vi "Save or Load Config.vi"(2 "GUI Helper Q":refnum<queue>, 4 "Config Select Ref":refnum<vi>, 5 "Auto Clust":refnum<vi>, 6 "Task Info in":refnum<vi>, 7 "Save?":bool, 8 "error in (no error)":errorcluster, 9 "Task Configuration Name":string, 10 "Task Selection in":refnum<vi>, 11 "GUI in":refnum<class "GUI.lvclass">) -> (0 "error out":errorcluster, 3 "GUI out":refnum<class "GUI.lvclass">)   [LabVIEW 2020, in "GUI.lvlib" / "GUI.lvclass"]
uses:
  GUI.lvclass
  Task selection df.ctl
  Task info df.ctl
  Automate df.ctl
  Task Active Enum df.ctl
  GUI.lvclass/GUI.ctl
  <vilib>/Utility/config.llb/NI_LVConfig.lvlib
panel:
  # "Patterns"
  # "Phase"
  # "Left        Right"
  # "Left        Right"
  # "Left Arm"
  # "Right Arm"
  # "Input Type"
  # "Task Type"
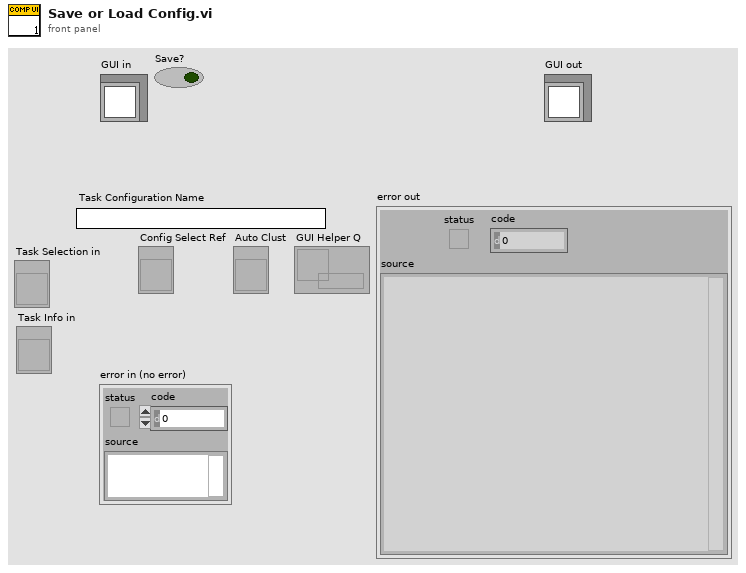
[diagram p1: front panel]
types:
  T1 = typedef "Task Active Enum df.ctl" = enum16{"Idle", "Start Freq Task", "Start Freq Task and Accel", "Start Scanning Task", "Start Scanning Task and Accel", "Preview Template", "Collect MVC", "Calibrate Force", "Calibrate Potentiometers", "Stop Helper", "EMG Mode", "EMG and Accel Mode", "Task Config Update"}
  T2 = typedef "NI_LVConfig.lvlib/Config Data RefNum.ctl" = refnum<k1>
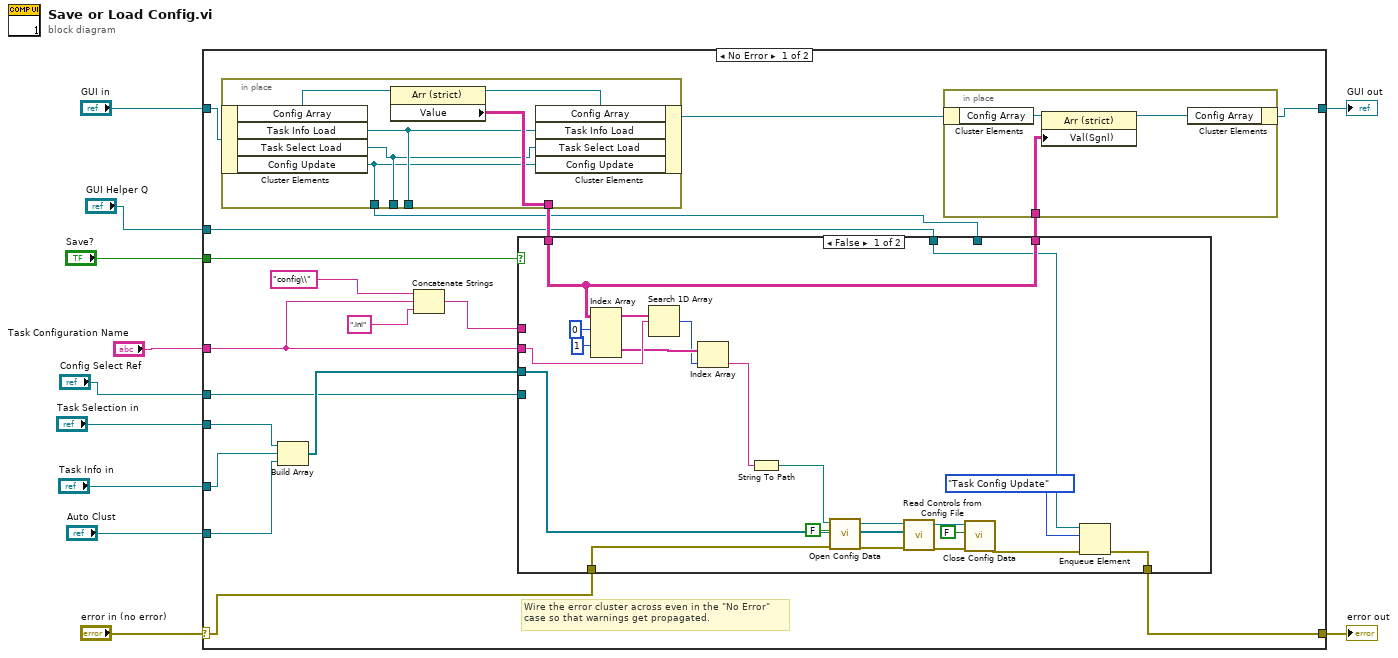
[diagram p0: block diagram]
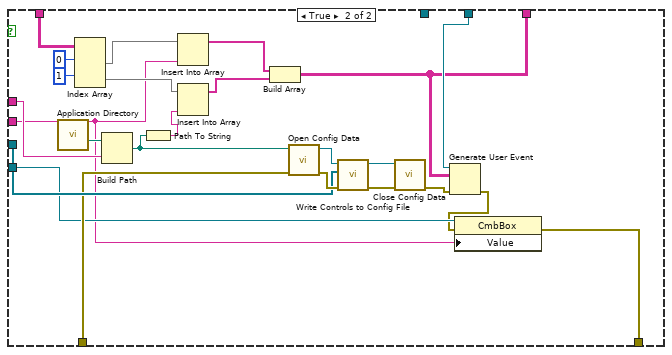
[diagram p2: hidden frame]
diagram:
  n1 = case shown="No Error" "error in (no error)" {
    selector: "error in (no error)" -> [w24 w86]
    tunnel: [w23 w86] -> w10
    tunnel: [w26 w85] -> w8
    tunnel: "GUI in" -> [w29 w85]
    tunnel: "Save?" -> [w30 _]
    tunnel: "Task Configuration Name" -> [w20 _]
    tunnel: "Task Selection in" -> [w18 _]
    tunnel: "Task Info in" -> [w17 _]
    tunnel: "Config Select Ref" -> [w14 _]
    tunnel: "Auto Clust" -> [w13 _]
    tunnel: "GUI Helper Q" -> [w12 _]
    frame No Error {
      # "Wire the error cluster across even in the \"No Error\"\ncase so that warnings get propagated."
      n2 = in-place {
        in-place-border: [w37] -> w28
        in-place-border: [w36] -> _
        in-place-border: [w35] -> _
        in-place-border: [w34] -> w16
        n3 = in-place-cluster #1(w29) -> ("Config Array"=w39:refnum<vi>, "Task Info Load"=w36:refnum<user-event>, "Task Select Load"=w35:refnum<user-event>, "Config Update"=w34:refnum<user-event>)
        n4 = property class="Arr (strict)"(reference=w39) -> (reference out=w38:refnum<vi>, "Value"=w37:string[][])  [unwired: 1 in, 1 out]
        n5 = in-place-cluster #1("Config Array"=w38, "Task Info Load"=w36, "Task Select Load"=w35, "Config Update"=w34) -> (w27:refnum<class "GUI.lvclass">)
      }
      n6 = Build Array(w18, w17, w13) -> (w19:refnum<vi>[])
      n7 = Concatenate Strings("config\\" ("string"), w20, ".ini" ("string")) -> (w21:string)
      n8 = case shown="False" w30 {
        tunnel: w19 -> [w53 w81]
        tunnel: w28 -> [w44 w75]
        tunnel: w20 -> [w49 w61]
        tunnel: [w44 w67] -> w25
        tunnel: w24 -> [w59 w80]
        tunnel: [w40 w62] -> w23
        tunnel: w21 -> [_ w70]
        tunnel: w16 -> [_ w77]
        tunnel: w14 -> [_ w64]
        tunnel: w12 -> [w43 _]
        frame False {
          n9 = Index Array(array=w44, index (row) #1=0 ("index (row)"), index (row) #2=1 ("index (row)")) -> (element #1=w50:string[], element #2=w48:string[])  [unwired: 2 in]
          n10 = Search 1D Array(1D array=w50, element=w49) -> (index of element=w47:i32)  [unwired: 1 in]
          n11 = Index Array(array=w48, index=w47) -> (element=w46:string)
          n12 = String To Path(string=w46) -> (path=w45:path)
          n13 = call <vilib>:"Open Config Data.vi"("error in (no error)"=w59, "create file if necessary (T)"=FALSE, "configuration file path"=w45) -> ("error out"=w57:errorcluster, "refnum"=w58:T2)  [unwired: 6 in, 1 out]
          n14 = call "Read Controls from Config File.vi"("error in (no error)"=w57, "Control References"=w53, "Configuration File Reference In"=w58) -> ("error out"=w54:errorcluster, "Configuration File Reference Out"=w56:T2)  [unwired: 7 in]
          n15 = call <vilib>:"Close Config Data.vi"("error in (no error)"=w54, "write file if changed (T)"=FALSE, "refnum"=w56) -> ("error out"=w42:errorcluster)  [unwired: 7 in, 1 out]
          n16 = Enqueue Element(queue=w43, element=Task_Active_Enum_df."Task Config Update", error in (no error)=w42) -> (error out=w40:errorcluster)  [unwired: 1 in, 2 out]
        }
        frame True {
          n17 = call <vilib>:"Application Directory.vi"() -> ("Application Directory"=w84:path)
          n18 = Index Array(array=w75, index (row) #1=0 ("index (row)"), index (row) #2=1 ("index (row)")) -> (element #1=w72:string[], element #2=w71:string[])  [unwired: 2 in]
          n19 = Build Path(base path=w84, name or relative path=w70) -> (appended path=w66:path)
          n20 = Path To String(path=w66) -> (string=w65:string)
          n21 = Insert Into Array(array=w72, new element=w61) -> (w69:string[])  [unwired: 1 in]
          n22 = Insert Into Array(array=w71, new element=w65) -> (w68:string[])  [unwired: 1 in]
          n23 = Build Array(w69, w68) -> (w67:string[][])
          n24 = call <vilib>:"Open Config Data.vi"("error in (no error)"=w80, "configuration file path"=w66) -> ("error out"=w83:errorcluster, "refnum"=w82:T2)  [unwired: 7 in, 1 out]
          n25 = call "Write Controls to Config File.vi"("error in (no error)"=w83, "Control References"=w81, "Configuration File Reference In"=w82) -> ("error out"=w79:errorcluster, "Configuration File Reference Out"=w78:T2)  [unwired: 7 in]
          n26 = call <vilib>:"Close Config Data.vi"("error in (no error)"=w79, "refnum"=w78) -> ("error out"=w76:errorcluster)  [unwired: 8 in, 1 out]
          n27 = Generate User Event(user event=w77, event data cluster=w67, error in=w76) -> (error out=w63:errorcluster)  [unwired: 1 in, 1 out]
          n28 = property class="CmbBox"(reference=w64, error in=w63, "Value"=w61) -> (error out=w62:errorcluster)  [unwired: 1 out]
        }
      }
      n29 = in-place {
        in-place-border: w25 -> [w31]
        n30 = in-place-cluster #2(w27) -> ("Config Array"=w33:refnum<vi>)
        n31 = property class="Arr (strict)"(reference=w33, "Val(Sgnl)"=w31) -> (reference out=w32:refnum<vi>)  [unwired: 1 in, 1 out]
        n32 = in-place-cluster #2("Config Array"=w32) -> (w26:refnum<class "GUI.lvclass">)
      }
    }
    frame Error {
    }
  }
  "error out" <- w10
  "GUI out" <- w8
